vi "RW Torque Output Loop.vi"() -> ()   [LabVIEW 2019, in "Part of Main VIs.lvlib" / "Torque Library.lvlib"]
uses:
  <vilib>/DAQmx/write.llb/DAQmx Write (Analog DBL 1Chan 1Samp).vi
  <extravilib>/ChannelInstances/Tag-bool/Read With Abort.vi
  <extravilib>/ChannelInstances/Tag-dbl/Write With Abort.vi
  <extravilib>/ChannelInstances/Tag-bool/Write With Abort.vi
  <extravilib>/ChannelInstances/Tag-dbl/Read With Abort.vi
  <extravilib>/ChannelInstances/Tag-bool/Instantiate.vi
  <extravilib>/ChannelInstances/Tag-dbl/Instantiate.vi
  <extravilib>/ChannelInstances/Tag-bool/Endpoint.vi
  <vilib>/DAQmx/create/channels.llb/DAQmx Create Channel (AO-Voltage-Basic).vi
  <extravilib>/ChannelInstances/Tag-dbl/EndpointRead.vi
  <vilib>/DAQmx/miscellaneous.llb/DAQmx Fill In Error Info.vi
  <extravilib>/ChannelInstances/Tag-bool/EndpointRead.vi
  <extravilib>/ChannelInstances/Tag-dbl/Endpoint.vi
  Torque Library.lvlib
  <resource>/objmgr/daqmx.rc
  <extravilib>/ChannelInstances/Tag-dbl.lvlib
  <extravilib>/ChannelInstances/Tag-bool.lvlib
panel:
  in  "stop":bool
  in  "String":string
  in  "Numeric":dbl
  out "Waveform Chart":waveform(dbl)(graph)
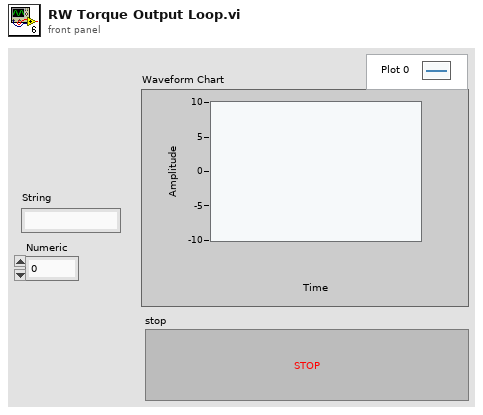
[diagram p1: front panel]
types:
  T1 = typedef "Tag-bool.lvlib/))Channel.ctl" = refnum<queue>
  T2 = typedef "Tag-dbl.lvlib/))Channel.ctl" = refnum<queue>
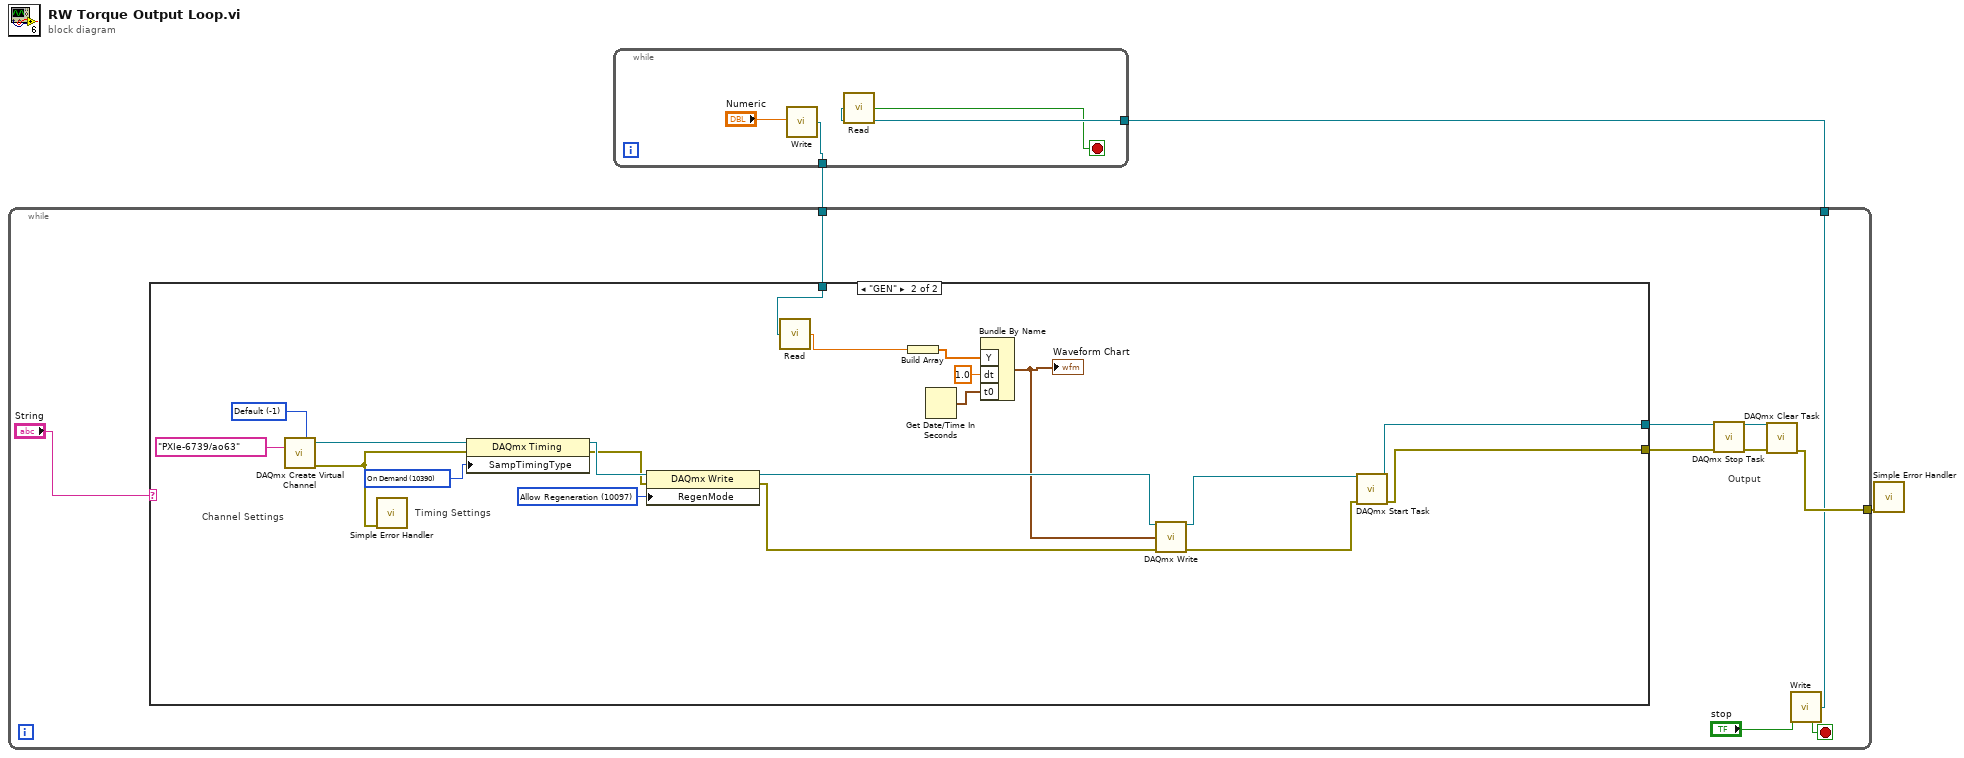
[diagram p0: block diagram]
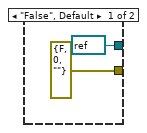
[diagram p2: hidden frame]
diagram:
  n1 = while {
    tunnel: [w7] -> w3
    tunnel: w2 -> [w6]
    tunnel: [w4] -> w1
    stop <- "stop" stop-if-true
    # "Output"
    n2 = case shown="\"GEN\"" "String" {
      tunnel: [refnum<k21> refnum ("task out") w26] -> w10
      tunnel: [errorcluster {"status"=FALSE, "code"=0, "source"=""} ("error out") w27] -> w9
      tunnel: w6 -> [_ w19]
      frame "False", Default {
      }
      frame "GEN" {
        w23 = 10097 items=["Allow Regeneration"=10097, "Do Not Allow Regeneration"=10158] ("RegenMode")
        w32 = 10390 items=["Sample Clock"=10388, "Burst Handshake"=12548, "Handshake"=10389, "Implicit"=10451, "On Demand"=10390, "Change Detection"=12504, "Pipelined Sample Clock"=14668] ("SampTimingType")
        w33 = -1 items=["Default"=-1, "RSE"=10083, "Differential"=10106, "Pseudodifferential"=12529] ("output terminal configuration")
        # "Timing Settings"
        # "Channel Settings"
        n3 = call-poly <vilib>:"DAQmx Create Virtual Channel.vi"("output terminal configuration"=w33, "physical channels"=tag "PXIe-6739/ao63") -> ("task out"=w31:refnum<k21>, "error out"=w30:errorcluster)  [unwired: 12 in]
        n4 = call <vilib>:"Simple Error Handler.vi"("error in (no error)"=w30) -> ()  [unwired: 4 in, 5 out]
        n5 = property class="DAQmx Timing"(reference=w31, error in=w30, "SampTimingType"=w32) -> (reference out=w25:refnum<k21>, error out=w24:errorcluster)
        n6 = property class="DAQmx Write"(reference=w25, error in=w24, "RegenMode"=w23) -> (reference out=w22:refnum<k21>, error out=w21:errorcluster)
        n7 = call <extravilib>:"Read.vi"("channel"=w19) -> ("element"=w18:dbl)  [unwired: 1 in, 1 out]
        n8 = Build Array(w18) -> (w17:dbl[])
        n9 = Get Date/Time In Seconds() -> (seconds since 1Jan1904=w20:timestamp)
        n10 = Bundle By Name("Y"=w17, "dt"=1.0, "t0"=w20) -> (w15:waveform(dbl))  [unwired: 1 in]
        "Waveform Chart" <- w15
        n11 = call-poly <vilib>:"DAQmx Write.vi"("task/channels in"=w22, "data"=w15, "error in"=w21) -> ("task out"=w29:refnum<k21>, "error out"=w28:errorcluster)  [unwired: 10 in, 1 out]
        n12 = call <vilib>:"DAQmx Start Task.vi"("task/channels in"=w29, "error in"=w28) -> ("task out"=w26:refnum<k21>, "error out"=w27:errorcluster)  [unwired: 12 in]
      }
    }
    n13 = call <vilib>:"DAQmx Stop Task.vi"("task/channels in"=w10, "error in"=w9) -> ("task out"=w11:refnum<k21>, "error out"=w12:errorcluster)  [unwired: 12 in]
    n14 = call <vilib>:"DAQmx Clear Task.vi"("task in"=w11, "error in"=w12) -> ("error out"=w7:errorcluster)  [unwired: 13 in]
    n15 = call <extravilib>:"Write.vi"("element"="stop") -> ("channel"=w4:T1)  [unwired: 1 out]
  }
  n16 = while {
    tunnel: [w37] -> w2
    tunnel: w1 -> [w36]
    stop <- w35 stop-if-true
    n17 = call <extravilib>:"Write.vi"("element"="Numeric") -> ("channel"=w37:T2)  [unwired: 1 out]
    n18 = call <extravilib>:"Read.vi"("channel"=w36) -> ("element"=w35:bool)  [unwired: 1 in, 1 out]
  }
  n19 = call <vilib>:"Simple Error Handler.vi"("error in (no error)"=w3) -> ()  [unwired: 4 in, 5 out]
